vi "Write Runtime Alias.vi"(8 "error in (no error)":errorcluster, 10 "Runtime Alias":string, 11 "Step Config in":refnum<class "Step Config.lvclass">) -> (0 "error out":errorcluster, 3 "Step Config out":refnum<class "Step Config.lvclass">)   [LabVIEW 2015, in "Step Config.lvclass"]
uses:
  Step Config.lvclass
  Step Config.lvclass/Step Config.ctl
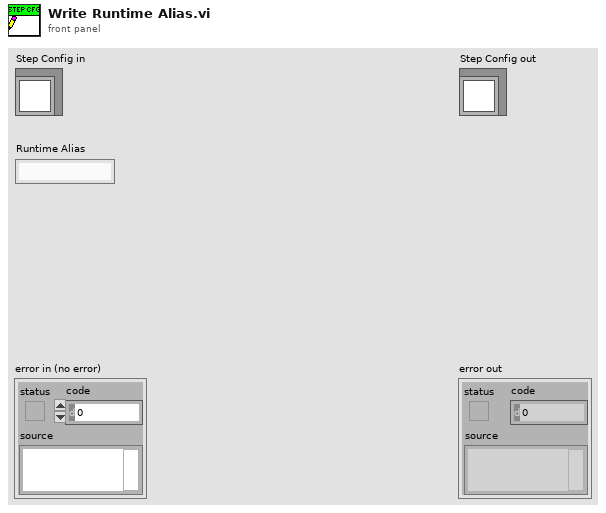
[diagram p1: front panel]
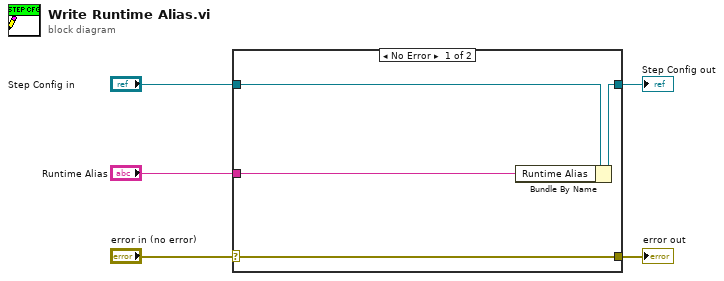
[diagram p0: block diagram]
diagram:
  n1 = case shown="No Error" "error in (no error)" {
    selector: "error in (no error)" -> [w9 w10]
    tunnel: [w9 w10] -> w4
    tunnel: [w7 w11] -> w2
    tunnel: "Step Config in" -> [w8 w11]
    tunnel: "Runtime Alias" -> [w6 _]
    frame No Error {
      n2 = Bundle By Name(cluster=w8, "Runtime Alias"=w6) -> (w7:refnum<class "Step Config.lvclass">)
    }
    frame Error {
    }
  }
  "error out" <- w4
  "Step Config out" <- w2
